vi "Set_Grating_Wavelength_txt.vi"(6 "Close VISA?":bool, 7 "file path (dialog if empty)":path=path "P:/inst/PrincetonInstruments - Acton/LabView/LVySpec GBL.txt", 8 "error in (no error)":errorcluster, 9 "Wavelength (nm)":dbl=780.0, 10 "Choose a grating":string(combo)="3", 11 "VISA resource name":refnum<visa-resource-name>="COM7") -> (0 "error out":errorcluster, 1 "Wavelength":string="?NM 779.991 nm  ", 2 "Grating being chosen":string="1200 BLZ=750 nm", 3 "VISA resource name out":refnum<visa-resource-name>="COM7")   [LabVIEW 2009]
uses:
  <vilib>/Utility/file.llb/Write To Spreadsheet File (DBL).vi
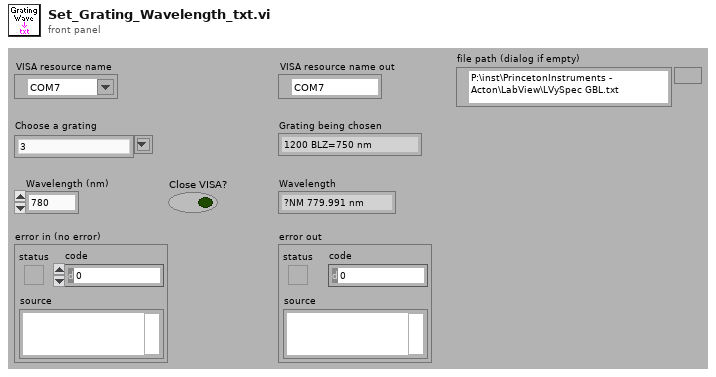
[diagram p1: front panel]
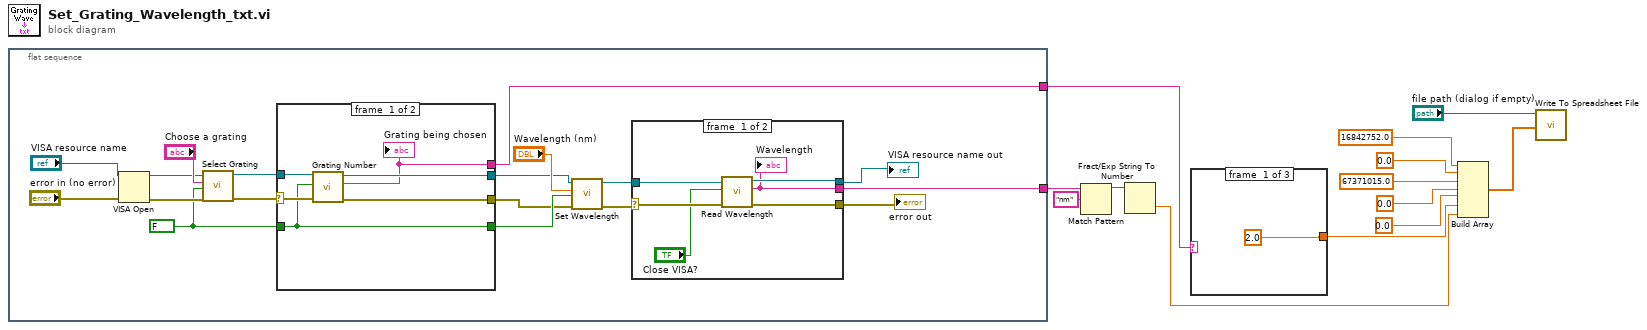
[diagram p0: block diagram]
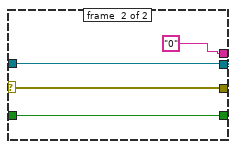
[diagram p2: hidden frame]
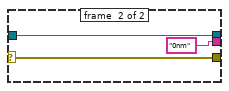
[diagram p3: hidden frame]
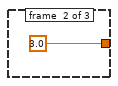
[diagram p4: hidden frame]
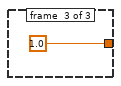
[diagram p5: hidden frame]
diagram:
  n1 = flat-sequence {
    tunnel: [w15] -> w5
    tunnel: [w14] -> w4
    frame #0 {
      w21 = FALSE ("Close VISA?")
      n2 = VISA Open(error in (no error)="error in (no error)", VISA resource name="VISA resource name") -> (VISA resource name=w23:refnum<visa-resource-name>, error out=w22:errorcluster)  [unwired: 3 out]
      n3 = call "Select Grating.vi"("error in (no error)"=w22, "Close VISA?"=w21, "Choose a grating"="Choose a grating", "VISA resource name"=w23) -> ("error out"=w25:errorcluster, "VISA resource name out"=w24:refnum<visa-resource-name>)  [unwired: 6 out]
      n4 = case shown="No Error" w25 {
        selector: w25 -> [w36 w40]
        tunnel: w24 -> [w37 w41]
        tunnel: w21 -> [w35 w39]
        tunnel: [w35 w39] -> w20
        tunnel: [w34 w41] -> w19
        tunnel: [w33 w40] -> w18
        tunnel: [w32 "0"] -> w15
        frame #0 {
          n5 = call "Grating Number.vi"("error in (no error)"=w36, "Close VISA?"=w35, "VISA resource name"=w37) -> ("error out"=w33:errorcluster, "Grating being chosen"=w32:string, "VISA resource name out"=w34:refnum<visa-resource-name>)  [unwired: 6 out]
          "Grating being chosen" <- w32
        }
        frame #1 {
        }
      }
      n6 = call "Set Wavelength.vi"("error in (no error)"=w18, "Close VISA?"=w20, "Wavelength (nm)"="Wavelength (nm)", "VISA resource name"=w19) -> ("error out"=w28:errorcluster, "VISA resource name out"=w27:refnum<visa-resource-name>)  [unwired: 6 out]
      n7 = case shown="No Error" w28 {
        selector: w28 -> [w47 w49]
        tunnel: w27 -> [w46 w50]
        tunnel: [w44 w50] -> w17
        tunnel: [w43 w49] -> w16
        tunnel: [w42 "0nm"] -> w14
        frame #0 {
          n8 = call "Read Wavelength.vi"("error in (no error)"=w47, "Close VISA?"="Close VISA?", "VISA resource name"=w46) -> ("error out"=w43:errorcluster, "Wavelength"=w42:string, "VISA resource name out"=w44:refnum<visa-resource-name>)  [unwired: 6 out]
          "Wavelength" <- w42
        }
        frame #1 {
        }
      }
      "VISA resource name out" <- w17
      "error out" <- w16
    }
  }
  n9 = Match Pattern(string=w4, regular expression="nm") -> (before substring=w2:string)  [unwired: 4 out]
  n10 = Fract/Exp String To Number(string=w2) -> (number=w1:dbl)  [unwired: 4 out]
  n11 = case shown="\"300 BLZ=750 nm\"" w5 {
    tunnel: [2.0 3.0 1.0] -> w9
    frame #0 {
    }
    frame #1 {
    }
    frame #2 {
    }
  }
  n12 = Build Array(16842752.0 ("Camera Handle"), 0.0 ("Spectrometer Handle"), 67371015.0 ("File Handle"), 0.0 ("Display Handle"), 0.0 ("Image Handle"), w9, w1) -> (w7:dbl[])
  n13 = call-poly <vilib>:"Write To Spreadsheet File.vi"("1D data"=w7, "file path (dialog if empty)"="file path (dialog if empty)") -> ()  [unwired: 4 in, 3 out]
